vi "send_motion_v1.vi"(8 "error in (no error)":errorcluster, 9 "Value in nm/u°":dbl, 10 "Axis":string(combo), 11 "IP address in":string="172.16.6.101") -> (0 "error out":errorcluster, 3 "IP address out":string="172.16.6.101")   [LabVIEW 2012]
panel:
  out "response":string
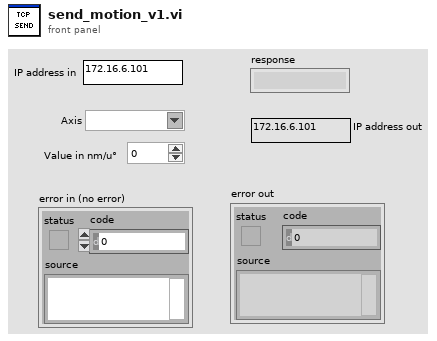
[diagram p1: front panel]
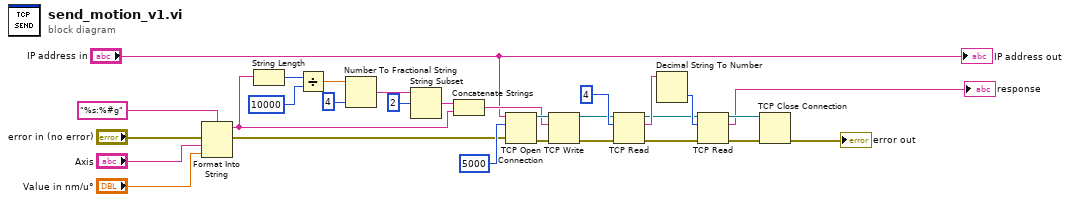
[diagram p0: block diagram]
diagram:
  n1 = Format Into String(format string="%s:%#g", error in="error in (no error)", "Axis", "Value in nm/u°") -> (resulting string=w27:string, error out=w7:errorcluster)  [unwired: 1 in]
  n2 = String Length(string=w27) -> (length=w23:i32)
  n3 = Divide(x=w23, y=10000) -> (x/y=w19:dbl)
  n4 = Number To Fractional String(number=w19, precision (6)=i16 4 ("Genauigkeit (6)")) -> (F-format string=w18:string)  [unwired: 2 in]
  n5 = String Subset(string=w18, offset (0)=2 ("Offset (0)")) -> (substring=w20:string)  [unwired: 1 in]
  n6 = Concatenate Strings(w20, w27) -> (w24:string)
  n7 = TCP Open Connection(address="IP address in", remote port or service name=u16 5000 ("Netzwerk-Port oder -Dienst"), error in (no error)=w7) -> (connection ID=w25:refnum<k5>, error out=w6:errorcluster)  [unwired: 2 in]
  n8 = TCP Write(connection ID=w25, data in=w24, error in (no error)=w6) -> (connection ID out=w12:refnum<k5>, error out=w5:errorcluster)  [unwired: 1 in, 1 out]
  n9 = TCP Read(connection ID=w12, bytes to read=4 ("Zu lesende Bytes"), error in (no error)=w5) -> (connection ID out=w13:refnum<k5>, data out=w15:string, error out=w4:errorcluster)  [unwired: 2 in]
  n10 = Decimal String To Number(string=w15) -> (number=w14:i32)  [unwired: 2 in, 1 out]
  n11 = TCP Read(connection ID=w13, bytes to read=w14, error in (no error)=w4) -> (connection ID out=w11:refnum<k5>, data out=→"response":string, error out=w3:errorcluster)  [unwired: 2 in]
  n12 = TCP Close Connection(connection ID=w11, error in (no error)=w3) -> (error out=→"error out":errorcluster)  [unwired: 1 in, 1 out]
  "IP address out" <- "IP address in"
